vi "F Inverse CDF.vi"(9 "k2":i32=1, 10 "k1":i32=2, 11 "cdf(x)":dbl=0.5) -> (0 "error":i32, 3 "x":dbl=1.5000000049999989)   [LabVIEW 2017, in "NI_Gmath.lvlib"]
doc: "Computes the continuous inverse cumulative distribution function (CDF) of the various distributions. You must manually select the polymorphic instance to use."
uses:
  <vilib>/gmath/NI_Gmath.lvlib
  <vilib>/gmath/statdist.llb/st_error_code.ctl
panel:
  # "F Inverse CDF"
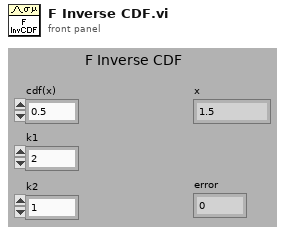
[diagram p1: front panel]
types:
  T1 = typedef "NI_Gmath.lvlib/st_error_code.ctl" = i32
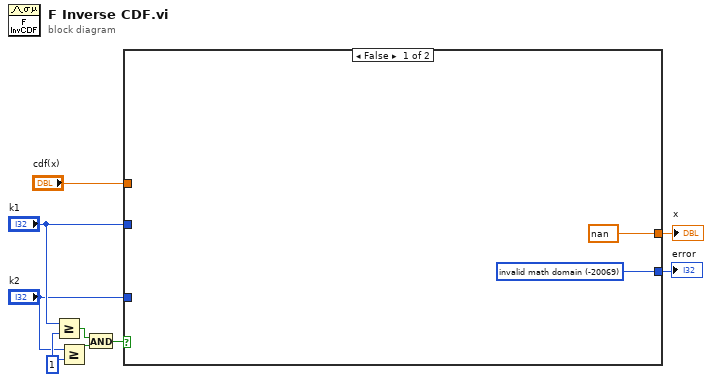
[diagram p0: block diagram]
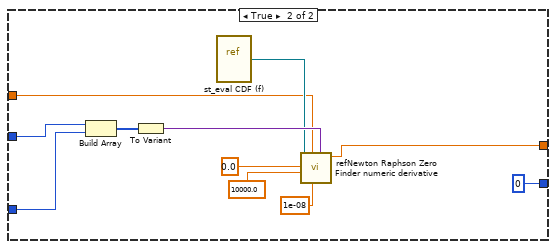
[diagram p2: hidden frame]
diagram:
  w2 = 1
  n1 = Greater Or Equal?(x="k1", y=w2) -> (x >= y?=w5:bool)
  n2 = Greater Or Equal?(x="k2", y=w2) -> (x >= y?=w6:bool)
  n3 = And(x=w5, y=w6) -> (x .and. y?=w3:bool)
  n4 = case shown="False" w3 {
    tunnel: "k2" -> [_ w19]
    tunnel: [w10 0 ("invalid math domain")] -> w9
    tunnel: [nan w15] -> w8
    tunnel: "cdf(x)" -> [_ w12]
    tunnel: "k1" -> [_ w20]
    frame False {
      w10 = T1 -20069 items=["invalid math domain"=-20069, "Fourier interpolation size m >= n"=-20070, "empty array"=-20003] ("stat interp error code")
    }
    frame True {
      n5 = Build Array(w20, w19) -> (w21:i32[])
      n6 = To Variant(anything=w21) -> (Variant=w14:variant)
      n7 = vi-ref <vilib>:"st_eval CDF (f).vi"() -> ("vi reference"=w13:refnum<vi>)
      n8 = call <vilib>:"refNewton Raphson Zero Finder numeric derivative.vi"("function parameters"=w14, "accuracy"=1e-08, "level"=w12, "end"=10000.0 ("upper limit"), "start"=0.0, "function refnum"=w13) -> ("zero"=w15:dbl)  [unwired: 2 in, 3 out]
    }
  }
  "x" <- w8
  "error" <- w9
